vi "Find Tags in Package.vi"(11 "Package":refnum<class "Package.lvclass">) -> (3 "Tags Front Matter":string)   [LabVIEW 2020]
doc: "This method loads the VIPMTag file on first call and uses it to find keywords in the Display Name and Description. When a keyword is found the cooresponding Tag is added to the Tag list."
uses:
  Libraries/Packages/Package_class/Package.lvclass
  Libraries/Packages/Package_class/Package.lvclass/Package.ctl
  Libraries/Packages/Package Version_class/Package Version.lvclass/Package Version.ctl
  Libraries/Packages/Package Version_class/Read Author.vi
  Libraries/Packages/Package Version_class/Read Dependencies.vi
  Libraries/Packages/Package Version_class/Read Description.vi
  Libraries/Packages/Package Version_class/Read DisplayName.vi
  Libraries/Packages/Package Version_class/Read Name.vi
  Libraries/Packages/Package Version_class/Read Release Notes.vi
  Libraries/Packages/Package Version_class/Read RepoName.vi
  Libraries/Packages/Package Version_class/Read Vendor.vi
  Libraries/Packages/Package Version_class/Read Summary.vi
  Libraries/Packages/Package_class/Read DisplayName.vi
  Libraries/Packages/Package_class/Read Name.vi
  Libraries/Packages/Package_class/Read RepoName.vi
  Libraries/Packages/Package_class/Read Versions.vi
  Libraries/Packages/Package Version_class/Package Version.lvclass
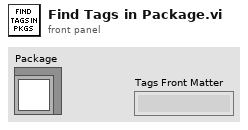
[diagram p1: front panel]
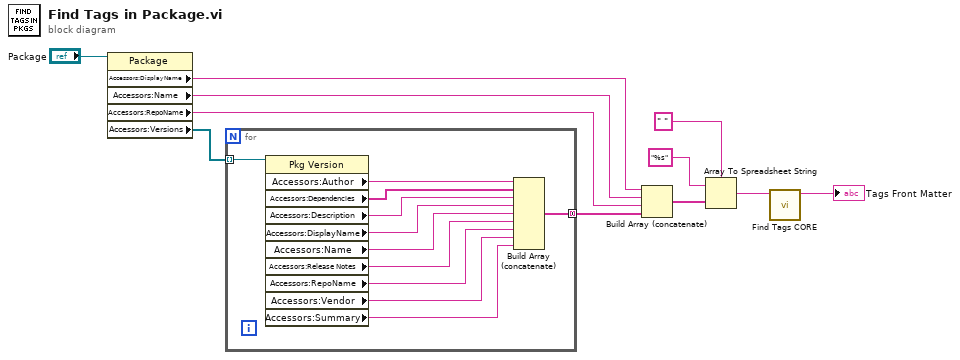
[diagram p0: block diagram]
diagram:
  n1 = property class="Package"(reference="Package") -> ("Accessors:DisplayName"=w9:string, "Accessors:Name"=w8:string, "Accessors:RepoName"=w7:string, "Accessors:Versions"=w10:refnum<class "Package Version.lvclass">[])  [unwired: 1 in, 2 out]
  n2 = for {
    tunnel: w10 -> [w22] mode=indexing
    tunnel: [w13] -> w6 mode=concatenating
    n3 = property class="Pkg Version"(reference=w22) -> ("Accessors:Author"=w21:string, "Accessors:Dependencies"=w20:string[], "Accessors:Description"=w19:string, "Accessors:DisplayName"=w18:string, "Accessors:Name"=w17:string, "Accessors:Release Notes"=w16:string, "Accessors:RepoName"=w15:string, "Accessors:Vendor"=w14:string, "Accessors:Summary"=w12:string)  [unwired: 1 in, 2 out]
    n4 = Build Array (concatenate)(w21, w20, w19, w18, w17, w16, w15, w14, w12) -> (w13:string[])
  }
  n5 = Build Array (concatenate)(w9, w8, w7, w6) -> (w5:string[])
  n6 = Array To Spreadsheet String(delimiter (Tab)=" ", array=w5, 3:"%s") -> (spreadsheet string=w2:string)
  n7 = call "Find Tags CORE.vi"("Index"=w2) -> ("Tags Front Matter"=→"Tags Front Matter":string)  [unwired: 10 in]
